vi "libssh2_knownhost_get.vi"(8 "error in (no error)":errorcluster, 10 "previous known host":T1, 11 "known hosts":T2) -> (0 "error out":errorcluster, 2 "next known host":T1, 3 "return value":i32)   [LabVIEW 2013, in "libssh2.lvlib"]
doc: "Gets a known host from the collection of known hosts."
uses:
  libssh2.lvlib
  Known Hosts Refnum.ctl
  Known Host Refnum.ctl
  libssh2.dll
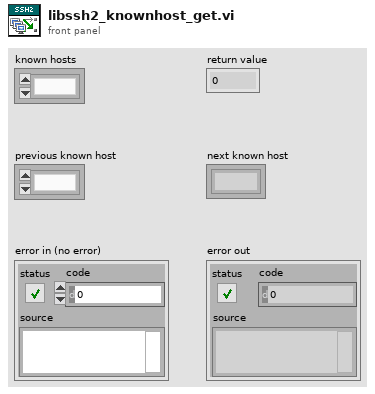
[diagram p1: front panel]
types:
  T1 = typedef "libssh2.lvlib/Known Host Refnum.ctl" = refnum<k1>
  T2 = typedef "libssh2.lvlib/Known Hosts Refnum.ctl" = refnum<k1>
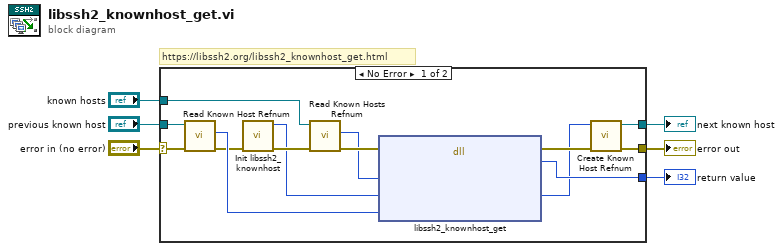
[diagram p0: block diagram]
diagram:
  # "https://libssh2.org/libssh2_knownhost_get.html"
  n1 = case shown="No Error" "error in (no error)" {
    selector: "error in (no error)" -> [w7 w21]
    tunnel: [w20 _] -> w6
    tunnel: [w18 w21] -> w5
    tunnel: "known hosts" -> [w16 _]
    tunnel: "previous known host" -> [w14 _]
    tunnel: [w12 _] -> w2
    frame No Error {
      n2 = call "Read Known Host Refnum.vi"("error in (no error)"=w7, "known host"=w14) -> ("error out"=w10:errorcluster, "libssh2_knownhost*"=w13:u64)  [unwired: 8 in]
      n3 = call "Init libssh2_knownhost.vi"("error in (no error)"=w10) -> ("error out"=w9:errorcluster, "libssh2_knownhost*"=w8:u64)  [unwired: 9 in]
      n4 = call "Read Known Hosts Refnum.vi"("error in (no error)"=w9, "known hosts"=w16) -> ("error out"=w17:errorcluster, "LIBSSH2_KNOWNHOSTS*"=w15:u64)  [unwired: 8 in]
      n5 = dll-call lib="C:/Users/pasca/source/repos/libssh2-labview/libssh2**.*" fn="libssh2_knownhost_get"(error in=w17, "hosts"=w15, "store"=w8, "prev"=w13) -> (error out=w19:errorcluster, "return value"=w20:i32, "store"=w11:u64)  [unwired: 4 in, 1 out]
      n6 = call "Create Known Host Refnum.vi"("error in (no error)"=w19, "libssh2_knownhost*"=w11) -> ("error out"=w18:errorcluster, "known host"=w12:T1)  [unwired: 8 in]
    }
    frame Error {
    }
  }
  "return value" <- w6
  "error out" <- w5
  "next known host" <- w2
